vi "ORS_GalvoConfig2D_uw.vi"(0 "Galvo":T1={"x mirror"="", "y mirror"="", "trig out"="", "x mirror task"="", "y mirror task"="", "trig out task"="", "n_axis"=0, "params"={"n_lines"=512, "n_frames"=1, "force to zero"=FALSE, "Triggers_per_sweep"=0.0, "X center"=0.0, "X span"=0.0, "Y center"=0.0, "Y span"=0.0, "flyb.lines"=0, "n_triggers"=0, "mode"=0, "offset"=5.0, "galvo phase"=0, "span factor"=1.0, "Custom trig."={"n_f to c. trig"=150, "c. trig length"=8, "c. trig interval"=1024, "n_c. trig"=1}, "f_per_pos"=1, "n_dataset"=1, "flyback fr"=1}, "acq trig out"="", "acq trig out task"="", "sample array X"=[], "sample array Y"=[], "custom trig out"="Dev1/port0/line7", "custom trig out task"="", "FDML-box"="TCPIP0::10.153.218.51::23::SOCKET", "ACQ/Galvo"=enum."ADC/FDML", "acq trig out an task"="", "acq trig out an"="", "Galvo Trig input"="", "Galvo Clk input"="", "sample array Acq trig out an"=[]} {"params"."n_dataset" min=1; "params"."X center" format="%^_3g"; "params"."X span" format="%^_3g"; "params"."Y center" format="%^_3g"; "params"."Y span" format="%^_3g"}, 3 "force to zero":bool, 5 "X center":dbl, 7 "X span":dbl=3.0, 9 "n_lines":i32=512, 11 "error in":errorcluster, 12 "Y center":dbl, 13 "Y span":dbl=3.0, 14 "Trigger-Murks-Faktor":dbl=1.0) -> (4 "Galvo out":T1={"x mirror"="", "y mirror"="", "trig out"="", "x mirror task"="", "y mirror task"="", "trig out task"="", "n_axis"=0, "params"={"n_lines"=512, "n_frames"=1, "force to zero"=FALSE, "Triggers_per_sweep"=0.0, "X center"=0.0, "X span"=0.0, "Y center"=0.0, "Y span"=0.0, "flyb.lines"=0, "n_triggers"=0, "mode"=0, "offset"=5.0, "galvo phase"=0, "span factor"=1.0, "Custom trig."={"n_f to c. trig"=150, "c. trig length"=8, "c. trig interval"=1024, "n_c. trig"=1}, "f_per_pos"=1, "n_dataset"=1, "flyback fr"=1}, "acq trig out"="", "acq trig out task"="", "sample array X"=[], "sample array Y"=[], "custom trig out"="Dev1/port0/line7", "custom trig out task"="", "FDML-box"="TCPIP0::10.153.218.51::23::SOCKET", "ACQ/Galvo"=enum."ADC/FDML", "acq trig out an task"="", "acq trig out an"="", "Galvo Trig input"="", "Galvo Clk input"="", "sample array Acq trig out an"=[]} {"params"."n_dataset" min=1; "params"."X center" format="%^_3g"; "params"."X span" format="%^_3g"; "params"."Y center" format="%^_3g"; "params"."Y span" format="%^_3g"}, 15 "error out":errorcluster)   [LabVIEW 2021]
uses:
  Typedefs/ORS_Galvo.ctl
  Typedefs/ORS_Galvo_params.ctl
  <vilib>/Analysis/1siggen.llb/Ramp Pattern by Samples.vi
  <vilib>/DAQmx/create/channels.llb/DAQmx Create Channel (AO-Voltage-Basic).vi
  <vilib>/Analysis/NI_AALBase.lvlib
  <resource>/objmgr/daqmx.rc
panel:
  out "sample array Acq trig out":dbl[](graph)
  out "sample array Y":dbl[](graph)
  out "sample array X":dbl[](graph)
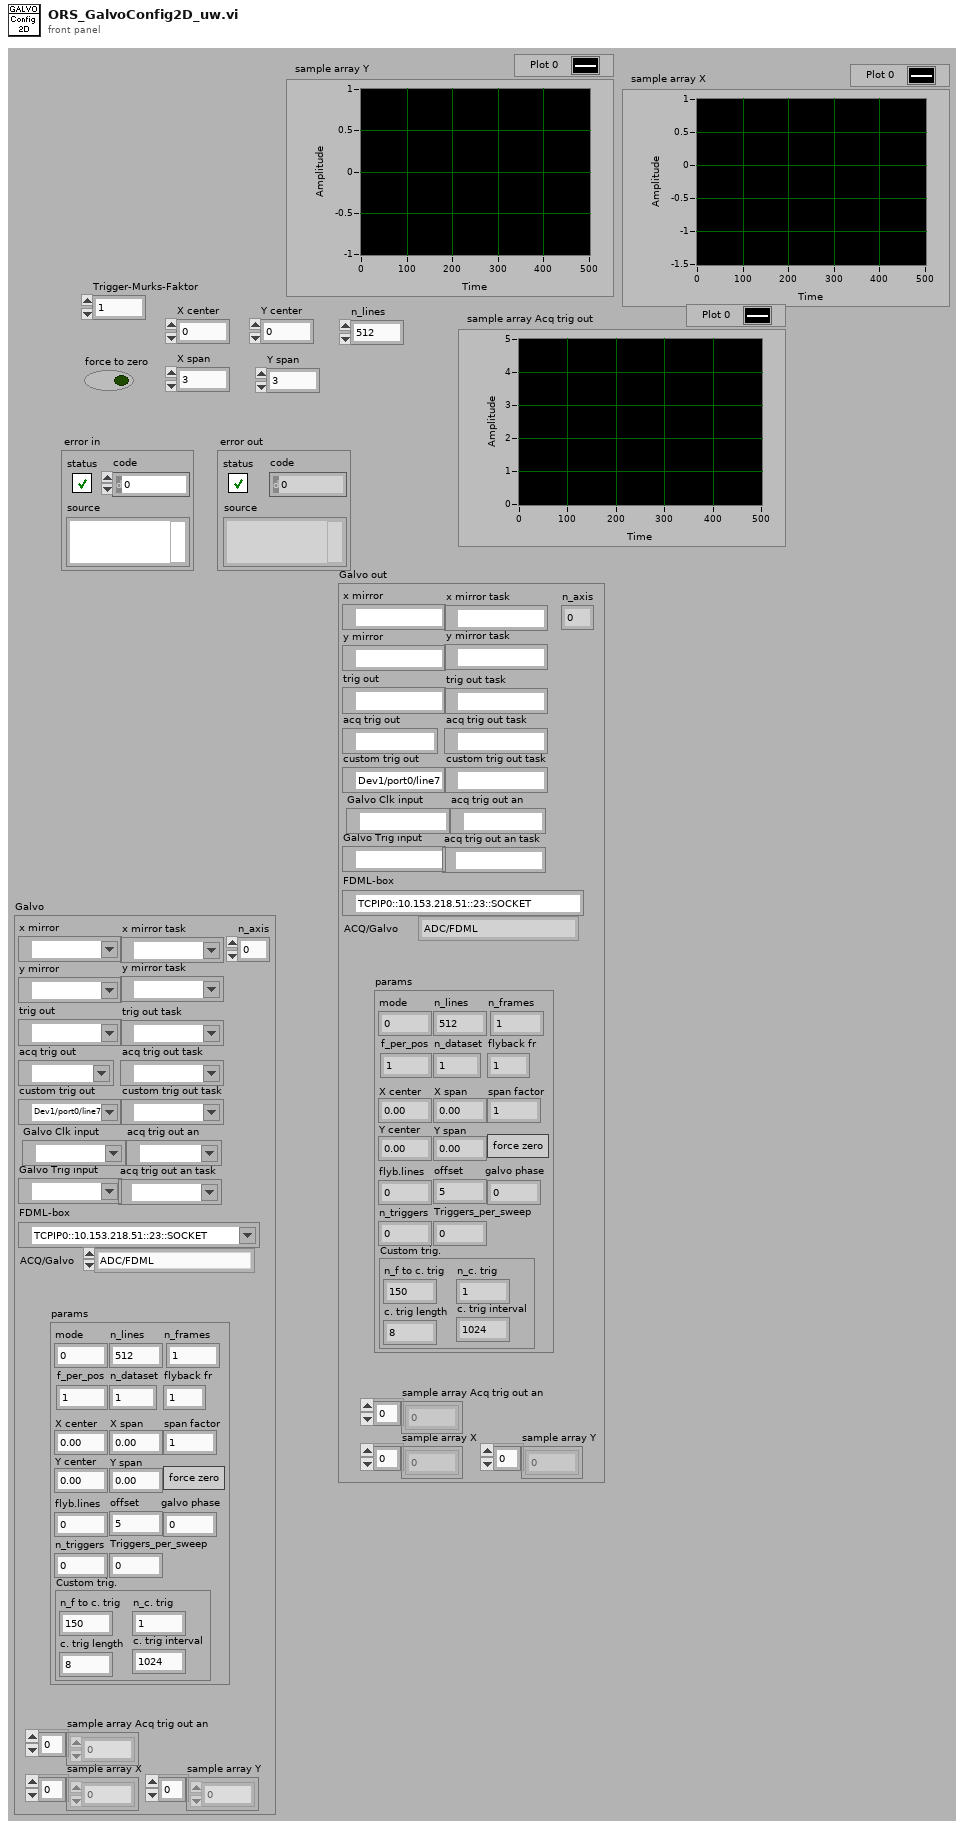
[diagram p1: front panel]
types:
  T1 = typedef "ORS_Galvo.ctl" = cluster{"x mirror":tag, "y mirror":tag, "trig out":tag, "x mirror task":refnum<k21>, "y mirror task":refnum<k21>, "trig out task":refnum<k21>, "n_axis":i32, "params":T2, "acq trig out":tag, "acq trig out task":refnum<k21>, "sample array X":dbl[], "sample array Y":dbl[], "custom trig out":tag, "custom trig out task":refnum<k21>, "FDML-box":refnum<visa-resource-name>, "ACQ/Galvo":enum16{"ADC/FDML", "NI_DAQ", "ADC"}, "acq trig out an task":refnum<k21>, "acq trig out an":tag, "Galvo Trig input":tag, "Galvo Clk input":tag, "sample array Acq trig out an":dbl[]}
  T2 = typedef "ORS_Galvo_params.ctl" = cluster{"n_lines":i32, "n_frames":i32, "force to zero":bool, "Triggers_per_sweep":dbl, "X center":dbl, "X span":dbl, "Y center":dbl, "Y span":dbl, "flyb.lines":i32, "n_triggers":i32, "mode":i32, "offset":dbl, "galvo phase":i32, "span factor":dbl, "Custom trig.":cluster{"n_f to c. trig":i32, "c. trig length":i32, "c. trig interval":i32, "n_c. trig":i32}, "f_per_pos":i32, "n_dataset":u32, "flyback fr":u16}
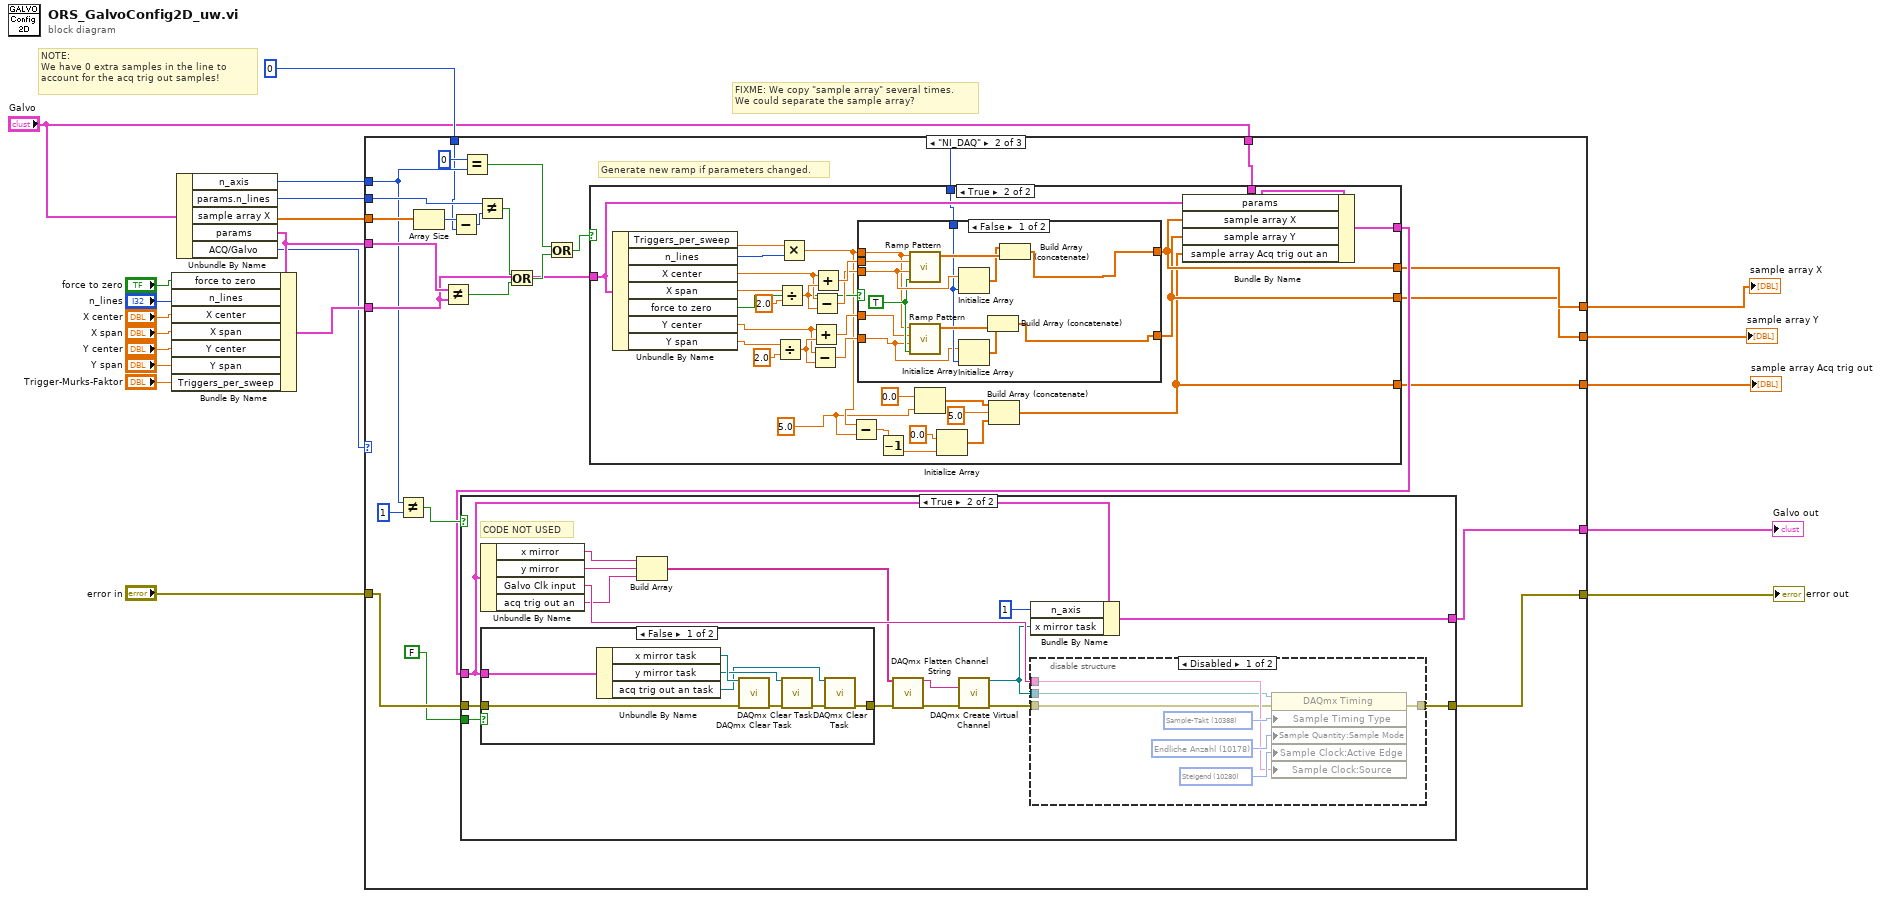
[diagram p0: block diagram]
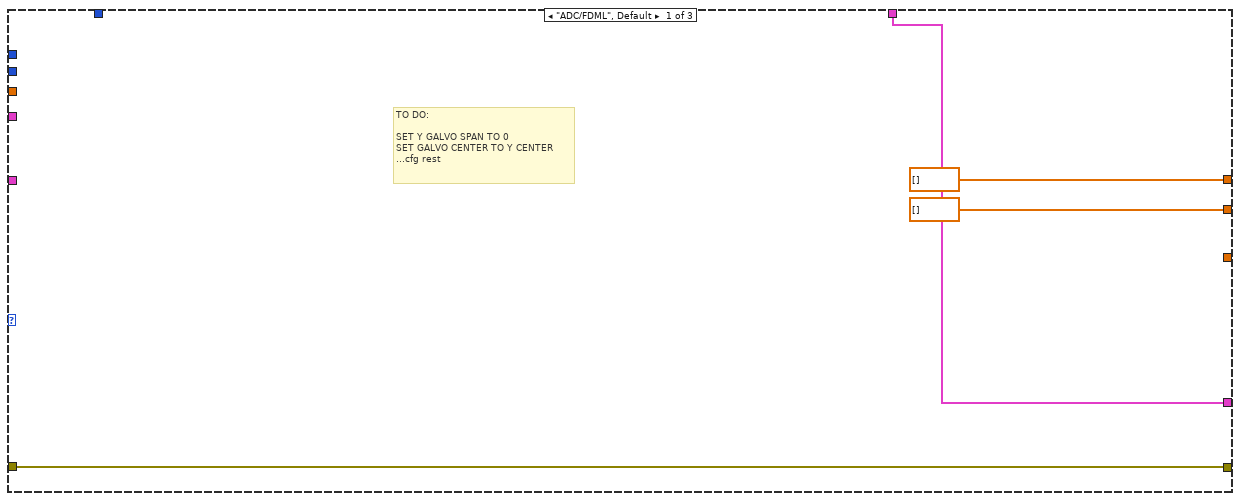
[diagram p2: hidden frame]
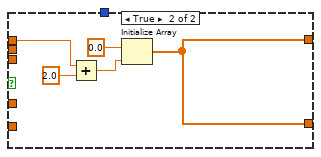
[diagram p7: hidden frame]
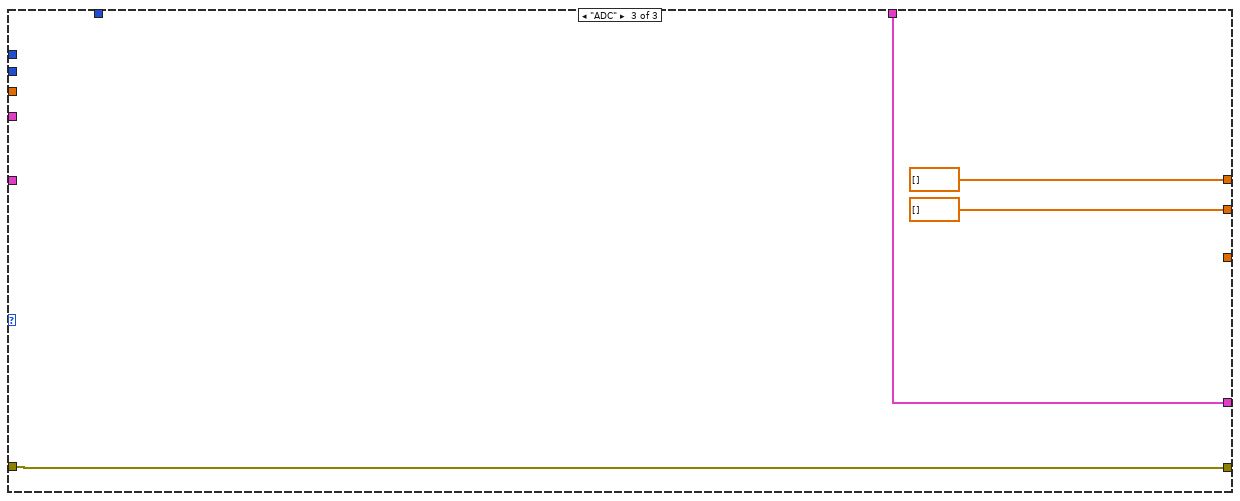
[diagram p8: hidden frame]
diagram:
  # "NOTE: \nWe have 0 extra samples in the line to \naccount for the acq trig out samples!"
  # "FIXME: We copy \"sample array\" several times. \nWe could separate the sample array?"
  n1 = Unbundle By Name("Galvo") -> ("n_axis"=w11:i32, "params.n_lines"=w13:i32, "sample array X"=w15:dbl[], "params"=w14:T2, "ACQ/Galvo"=w2:enum16{"ADC/FDML", "NI_DAQ", "ADC"})
  n2 = Bundle By Name(cluster=w14, "force to zero"="force to zero", "n_lines"="n_lines", "X center"="X center", "X span"="X span", "Y center"="Y center", "Y span"="Y span", "Triggers_per_sweep"="Trigger-Murks-Faktor") -> (w12:T2)
  n3 = case shown="\"NI_DAQ\"" w2 {
    tunnel: "error in" -> [w22 w50 w137]
    tunnel: w15 -> [_ w49 _]
    tunnel: w14 -> [_ w48 _]
    tunnel: w13 -> [_ w47 _]
    tunnel: w12 -> [_ w41 _]
    tunnel: w11 -> [_ w40 _]
    tunnel: [w22 w36 w137] -> w10
    tunnel: 0 ("y") -> [_ w31 _]
    tunnel: "Galvo" -> [w23 w30 w138]
    tunnel: [w23 w29 w138] -> w5
    tunnel: [dbl[] [] w28 dbl[] []] -> w4
    tunnel: [dbl[] [] w27 dbl[] []] -> w3
    tunnel: [_ w26 _] -> w1
    frame "ADC/FDML", Default {
      # "TO DO:\n\nSET Y GALVO SPAN TO 0\nSET GALVO CENTER TO Y CENTER\n...cfg rest"
    }
    frame "NI_DAQ" {
      # "Generate new ramp if parameters changed."
      n4 = Not Equal?(x=w40, y=1 ("x")) -> (x != y?=w38:bool)
      n5 = Array Size(array=w49) -> (size(s)=w32:i32)
      n6 = Not Equal?(x=w48, y=w41) -> (x != y?=w46:bool)
      n7 = Subtract(x=w32, y=w31) -> (x-y=w33:i32)
      n8 = Equal?(x=0, y=w40) -> (x = y?=w35:bool)
      n9 = Not Equal?(x=w47, y=w33) -> (x != y?=w44:bool)
      n10 = Or(x=w44, y=w46) -> (x .or. y?=w45:bool)
      n11 = Or(x=w35, y=w45) -> (x .or. y?=w42:bool)
      n12 = case shown="True" w42 {
        tunnel: w41 -> [_ w105]
        tunnel: w30 -> [w85 w107]
        tunnel: [w85 w106] -> w37
        tunnel: w31 -> [_ w104]
        tunnel: [_ w97] -> w28
        tunnel: [_ w96] -> w27
        tunnel: [_ w93] -> w26
        frame False {
        }
        frame True {
          w90 = 5.0
          n13 = Unbundle By Name(w105) -> ("Triggers_per_sweep"=w110:dbl, "n_lines"=w108:i32, "X center"=w112:dbl, "X span"=w111:dbl, "force to zero"=w109:bool, "Y center"=w101:dbl, "Y span"=w100:dbl)
          n14 = Divide(x=w100, y=2.0) -> (x/y=w103:dbl)
          n15 = Divide(x=w111, y=2.0) -> (x/y=w115:dbl)
          n16 = Multiply(x=w110, y=w108) -> (x*y=w91:dbl)
          n17 = Subtract(x=w101, y=w103) -> (x-y=w98:dbl)
          n18 = Add(x=w101, y=w103) -> (x+y=w99:dbl)
          n19 = Subtract(x=w112, y=w115) -> (x-y=w113:dbl)
          n20 = Add(x=w112, y=w115) -> (x+y=w114:dbl)
          n21 = Subtract(x=w91, y=w90) -> (x-y=w88:dbl)
          n22 = case shown="False" w109 {
            tunnel: [w118 w130] -> w97
            tunnel: w114 -> [w129 _]
            tunnel: w113 -> [w126 _]
            tunnel: w91 -> [w121 w132]
            tunnel: w104 -> [w122 _]
            tunnel: [w117 w130] -> w96
            tunnel: w99 -> [w120 _]
            tunnel: w98 -> [w119 _]
            frame False {
              w123 = TRUE ("exclude end?")
              n23 = call-poly <vilib>:"Ramp Pattern.vi"("exclude end?"=w123, "start"=w126, "end"=w129, "samples"=w121) -> ("Ramp Pattern"=w128:dbl[])  [unwired: 6 in, 1 out]
              n24 = call-poly <vilib>:"Ramp Pattern.vi"("exclude end?"=w123, "start"=w119, "end"=w120, "samples"=w121) -> ("Ramp Pattern"=w124:dbl[])  [unwired: 6 in, 1 out]
              n25 = Initialize Array(w126, w122) -> (w127:dbl[])
              n26 = Initialize Array(w119, w122) -> (w125:dbl[])
              n27 = Build Array (concatenate)(w125, w124) -> (w117:dbl[])
              n28 = Build Array (concatenate)(w127, w128) -> (w118:dbl[])
            }
            frame True {
              n29 = Add(x=w132, y=2.0) -> (x+y=w133:dbl)
              n30 = Initialize Array(0.0 ("element"), w133) -> (w130:dbl[])
            }
          }
          n31 = Decrement(x=w88) -> (x-1=w89:dbl)
          n32 = Initialize Array(0.0 ("element"), w90) -> (w87:dbl[])
          n33 = Initialize Array(0.0 ("element"), w89) -> (w94:dbl[])
          n34 = Build Array (concatenate)(w87, 5.0 ("element"), w94) -> (w93:dbl[])
          n35 = Bundle By Name(cluster=w107, "params"=w105, "sample array X"=w97, "sample array Y"=w96, "sample array Acq trig out an"=w93) -> (w106:T1)
        }
      }
      n36 = case shown="True" w38 {
        tunnel: w50 -> [w52 w63]
        tunnel: w37 -> [w51 w64]
        tunnel: [w52 w67] -> w36
        tunnel: [w51 w66] -> w29
        tunnel: FALSE -> [_ w65]
        frame False {
        }
        frame True {
          # "CODE NOT USED"
          n37 = Unbundle By Name(w64) -> ("x mirror"=w58:tag, "y mirror"=w57:tag, "Galvo Clk input"=w68:tag, "acq trig out an"=w53:tag)
          n38 = case shown="False" w65 {
            tunnel: w64 -> [w81 _]
            tunnel: w63 -> [w80 w84]
            tunnel: [w76 w84] -> w56
            frame False {
              n39 = Unbundle By Name(w81) -> ("x mirror task"=w83:refnum<k21>, "y mirror task"=w82:refnum<k21>, "acq trig out an task"=w78:refnum<k21>)
              n40 = call <vilib>:"DAQmx Clear Task.vi"("task in"=w83, "error in"=w80) -> ("error out"=w79:errorcluster)  [unwired: 13 in]
              n41 = call <vilib>:"DAQmx Clear Task.vi"("task in"=w82, "error in"=w79) -> ("error out"=w77:errorcluster)  [unwired: 13 in]
              n42 = call <vilib>:"DAQmx Clear Task.vi"("task in"=w78, "error in"=w77) -> ("error out"=w76:errorcluster)  [unwired: 13 in]
            }
            frame True {
            }
          }
          n43 = Build Array(w58, w57, w53) -> (w59:tag[])
          n44 = call <vilib>:"DAQmx Flatten Channel String.vi"("names in"=w59, "error in"=w56) -> ("names out"=w60:string, "error out"=w61:errorcluster)  [unwired: 12 in]
          n45 = call-poly <vilib>:"DAQmx Create Virtual Channel.vi"("physical channels"=w60, "error in"=w61) -> ("task out"=w54:refnum<k21>, "error out"=w55:errorcluster)  [unwired: 12 in]
          n46 = Bundle By Name(cluster=w64, "n_axis"=1, "x mirror task"=w54) -> (w66:T1)
          n47 = disable-structure shown="Disabled" {
            disable-tunnel: w68 -> [w72 _]
            disable-tunnel: [w71 _] -> w67
            disable-tunnel: w55 -> [w70 _]
            disable-tunnel: w54 -> [w69 _]
            frame Disabled {
              w75 = 10280 items=["Steigend"=10280, "Fallend"=10171] ("SampleTakt.AktiveFlanke")
              w74 = 10178 items=["Endliche Anzahl"=10178, "kontinuierlich"=10123, "Einzelwert (HW-getaktet)"=12522] ("SampleAnzahl.SampleModus")
              w73 = 10388 items=["Sample-Takt"=10388, "Burst-Handshake"=12548, "Handshake"=10389, "implizit"=10451, "1 Sample"=10390, "Änderungserkennung"=12504, "Sample-Takt in Pipeline"=14668] ("SampleTimingArt")
              n48 = property class="DAQmx Timing"(reference=w69, error in=w70, "Sample Timing Type"=w73, "Sample Quantity:Sample Mode"=w74, "Sample Clock:Active Edge"=w75, "Sample Clock:Source"=w72) -> (error out=w71:errorcluster)  [unwired: 1 out]
            }
            frame Enabled {
            }
          }
        }
      }
    }
    frame "ADC" {
    }
  }
  "error out" <- w10
  "Galvo out" <- w5
  "sample array X" <- w4
  "sample array Y" <- w3
  "sample array Acq trig out" <- w1
